vi "WriteChannel Name.vi"(8 "Error In":errorcluster, 10 "Channel Name":string="ch0", 11 "object in":refnum<class "AW Config.lvclass">) -> (0 "Error Out":errorcluster, 3 "object out":refnum<class "AW Config.lvclass">)   [LabVIEW 2023, in "PXI-5441.lvlib" / "AW Config.lvclass"]
uses:
  AW Config.lvclass
  AW Config.lvclass/AW Config.ctl
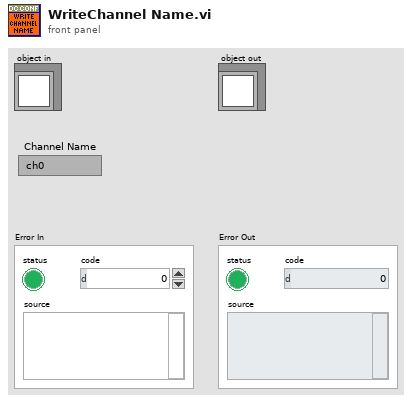
[diagram p1: front panel]
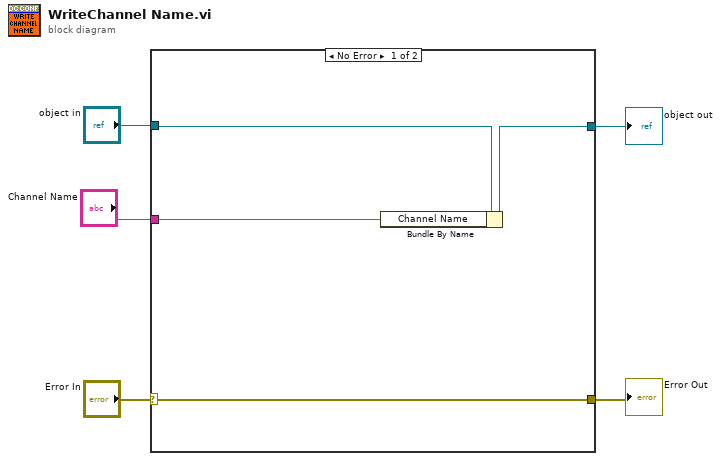
[diagram p0: block diagram]
diagram:
  n1 = case shown="No Error" "Error In" {
    selector: "Error In" -> [w8 w11]
    tunnel: [w8 w11] -> w4
    tunnel: [w6 w10] -> w2
    tunnel: "object in" -> [w7 w10]
    tunnel: "Channel Name" -> [w9 _]
    frame No Error {
      n2 = Bundle By Name(cluster=w7, "Channel Name"=w9) -> (w6:refnum<class "AW Config.lvclass">)
    }
    frame Error {
    }
  }
  "Error Out" <- w4
  "object out" <- w2
